vi "3D display.vi"(0 "Camera Position":T1={"X"=3000.0, "Y"=0.0, "Z"=1000.0}, 1 "Scene in":refnum<vi>, 2 "Target":T1, 3 "Up Direction":T1={"X"=0.0, "Y"=0.0, "Z"=1.0}, 4 "Reset camera":bool) -> (5 "3D Picture":refnum<vi>(3d-picture))   [LabVIEW 2018]
uses:
  <vilib>/Utility/miscctls.llb/LV3DPointTypeDef.ctl
  Collision Detection global.vi
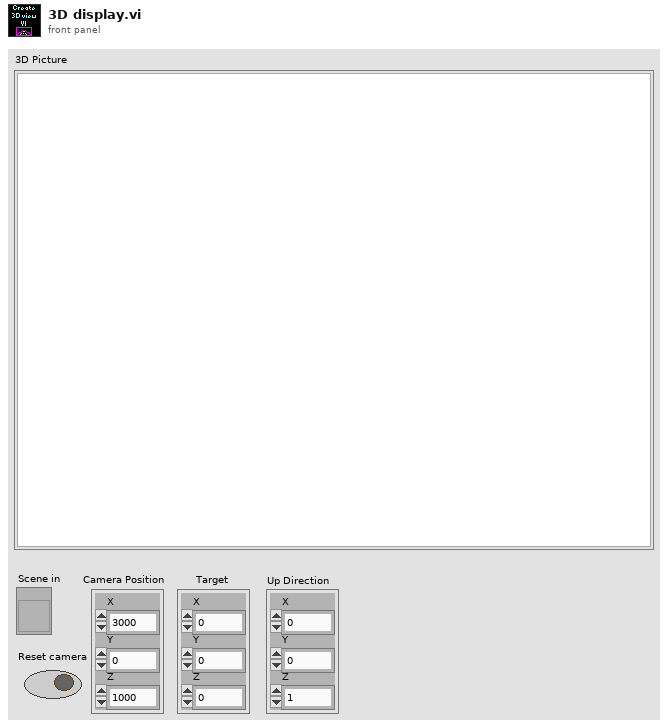
[diagram p1: front panel]
types:
  T1 = typedef "LV3DPointTypeDef.ctl" = cluster{"X":sgl, "Y":sgl, "Z":sgl}
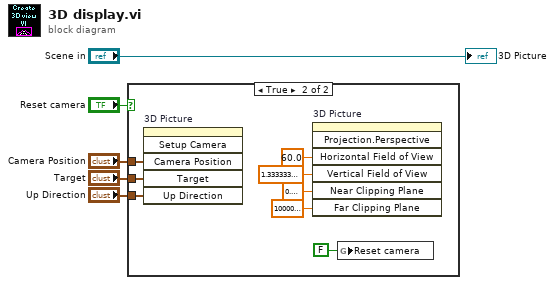
[diagram p0: block diagram]
diagram:
  n1 = case shown="True" "Reset camera" {
    tunnel: "Camera Position" -> [_ w9]
    tunnel: "Target" -> [_ w8]
    tunnel: "Up Direction" -> [_ w7]
    frame False {
    }
    frame True {
      n2 = invoke on="3D Picture" class="SceneGraphDisp (strict)" method="Setup Camera"("Camera Position"=w9, "Target"=w8, "Up Direction"=w7) -> ()  [unwired: 3 in, 6 out]
      n3 = invoke on="3D Picture" class="SceneGraphDisp (strict)" method="Projection.Perspective"("Horizontal Field of View"=sgl 60.0 ("Field of View"), "Vertical Field of View"=sgl 1.3333334 ("Aspect Ratio"), "Near Clipping Plane"=sgl 0.1, "Far Clipping Plane"=sgl 1000000.0) -> ()  [unwired: 3 in, 7 out]
      n4 = global write "Collision Detection global.vi" "Reset camera"(FALSE ("Reset camera")) -> ()
    }
  }
  "3D Picture" <- "Scene in"
